vi "AppendToLogFile.vi"(9 "text":string, 11 "DumpFile":path) -> ()   [LabVIEW 2024]
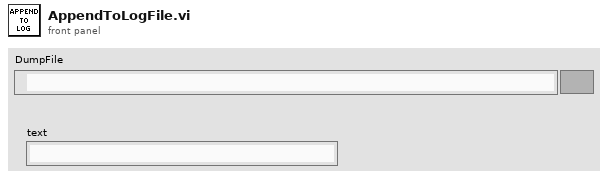
[diagram p1: front panel]
types:
  T1 = enum16{"open", "replace", "create", "open or create", "replace or create", "replace or create with confirmation"}
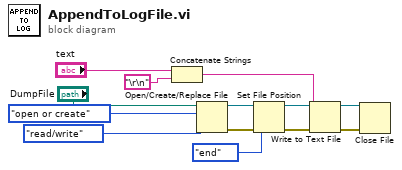
[diagram p0: block diagram]
diagram:
  n1 = Concatenate Strings("text", "\r\n") -> (w2:string)
  n2 = Open/Create/Replace File(file path (use dialog)="DumpFile", operation (0:open)=T1."open or create", access (0:read/write)=enum16{"read/write", "read-only", "write-only"}."read/write") -> (refnum out=w9:refnum<file>, error out=w10:errorcluster)  [unwired: 3 in, 1 out]
  n3 = Set File Position(refnum=w9, from (0:start)=enum16{"start", "end", "current"}."end", error in=w10) -> (refnum out=w7:refnum<file>, error out=w6:errorcluster)  [unwired: 1 in]
  n4 = Write to Text File(file (use dialog)=w7, text=w2, error in=w6) -> (refnum out=w3:refnum<file>, error out=w4:errorcluster)  [unwired: 1 in, 1 out]
  n5 = Close File(refnum=w3, error in=w4) -> ()  [unwired: 2 out]
